vi "ControlValueSave.vi"(6 "ファイル名入力?(f)":bool, 8 "err(in)":errorcluster, 11 "VI refnum":refnum<vi>) -> (0 "err(out)":errorcluster)   [LabVIEW 2016]
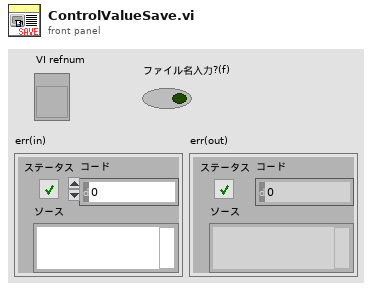
[diagram p1: front panel]
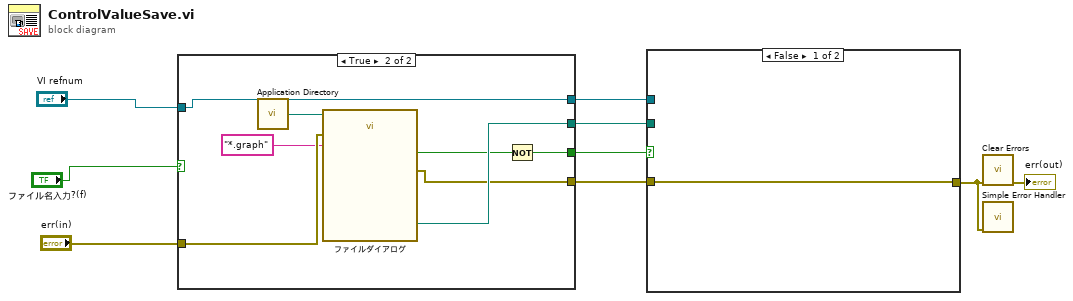
[diagram p0: block diagram]
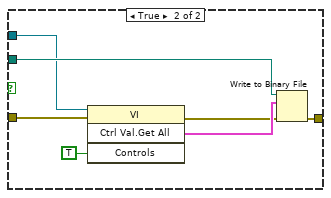
[diagram p2: hidden frame]
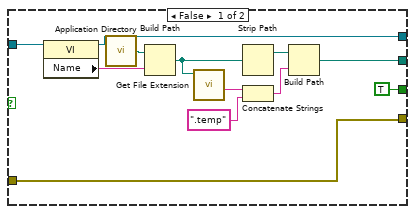
[diagram p3: hidden frame]
diagram:
  n1 = case shown="TRUE" "ファイル名入力?(f)" {
    tunnel: [w21 w29] -> w7
    tunnel: "VI refnum" -> [w20 w28]
    tunnel: [w19 w28] -> w5
    tunnel: [w11 w27] -> w2
    tunnel: "err(in)" -> [w11 w26]
    tunnel: [TRUE w24] -> w1
    frame False {
      n2 = property class="VI"(reference=w20) -> (reference out=w19:refnum<vi>, "Name"=w17:string)  [unwired: 1 in, 1 out]
      n3 = call <vilib>:"Application Directory.vi"() -> ("Application Directory"=w18:path)
      n4 = Build Path(base path=w18, name or relative path=w17) -> (appended path=w12:path)
      n5 = call <vilib>:"Get File Extension.vi"("file"=w12) -> ("filename without extension"=w15:string)  [unwired: 6 in, 4 out]
      n6 = Strip Path(path=w12) -> (stripped path=w16:path)  [unwired: 1 out]
      n7 = Concatenate Strings(w15, ".temp" ("名前または相対パス")) -> (w13:string)
      n8 = Build Path(base path=w16, name or relative path=w13) -> (appended path=w21:path)
    }
    frame True {
      n9 = call <vilib>:"Application Directory.vi"() -> ("Application Directory"=w22:path)
      n10 = call "ファイルダイアログ"("start path"=w22, "error in"=w26, "pattern (all files)"="*.graph") -> ("selected path"=w29:path, "cancelled"=w25:bool, "error out"=w27:errorcluster)  [unwired: 9 in, 1 out]
      n11 = Not(x=w25) -> (.not. x?=w24:bool)
    }
  }
  n12 = case shown="FALSE" w1 {
    tunnel: [w30 w37] -> w8
    tunnel: w7 -> [_ w36]
    tunnel: w5 -> [_ w35]
    tunnel: w2 -> [w30 w31]
    frame False {
    }
    frame True {
      n13 = invoke class="VI" method="Ctrl Val.Get All"(reference=w35, error in=w31, "Controls"=TRUE ("制御器")) -> (error out=w32:errorcluster, "Get All Control Values Variant"=w33:cluster{"Name":string, "Variant Data":variant}[])  [unwired: 1 in, 2 out]
      n14 = Write to Binary File(file (use dialog)=w36, data=w33, error in=w32) -> (error out=w37:errorcluster)  [unwired: 3 in, 2 out]
    }
  }
  n15 = call <vilib>:"Clear Errors.vi"("error in (no error)"=w8) -> ("error out"=→"err(out)":errorcluster)  [unwired: 5 in, 1 out]
  n16 = call <vilib>:"Simple Error Handler.vi"("error in (no error)"=w8) -> ()  [unwired: 4 in, 5 out]
